vi "Monitor_Cliente_Consumidor.vi"() -> ()   [LabVIEW 2024]
uses:
  controls/Oven.ctl
  controls/Acquire.ctl
panel:
  out "# elements in queue":i32
  out "Temp Acq":string="View Acquired Data"
  out "State control":string="View Acquired Data"
  out "Ventilator":bool
  in  "User Control":T1
  out "Historic Data":T2
  out "Heater Lebel [V]":dbl
  in  "Quit":bool
  in  "Stop Acq":bool
  in  "Start Acq":bool
  out "Temp. Display":T3(graph)
  out "Temp [ºC]":dbl(slide) scale=0.0..100.0
  out "HEATER":string
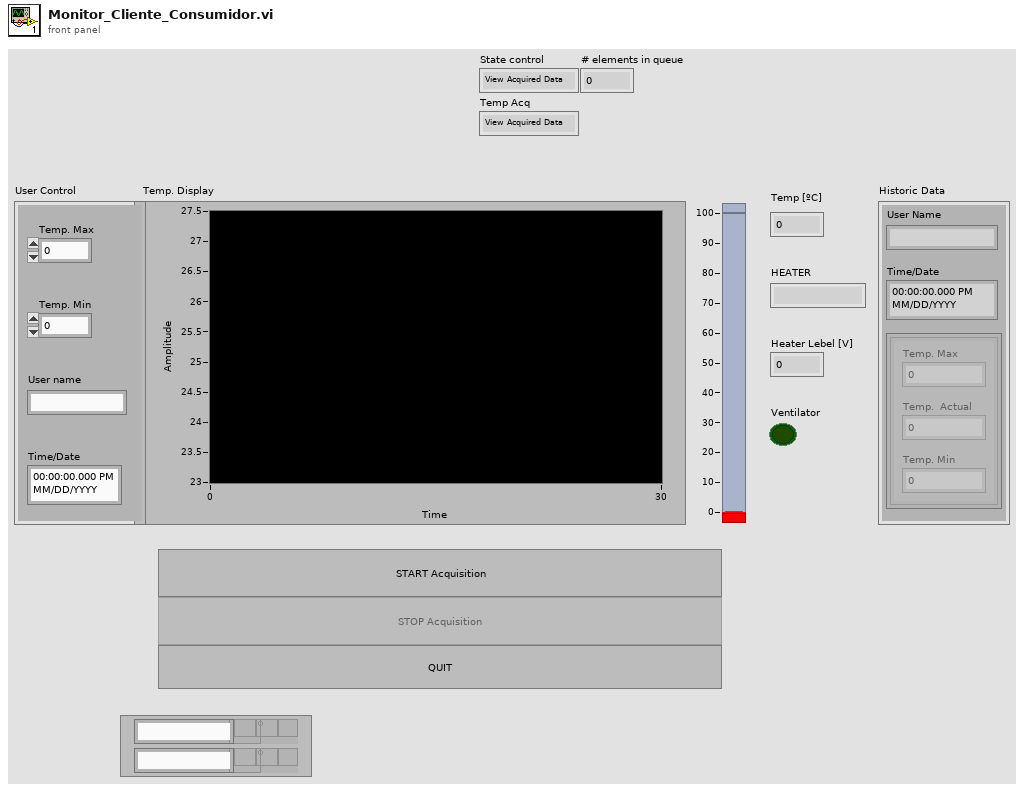
[diagram p1: front panel]
types:
  T1 = cluster{"Temp. Max":dbl, "Temp. Min":dbl, "User name":string, "Time/Date":timestamp}
  T2 = cluster{"User Name":string, "Time/Date":timestamp, "Array":cluster{"Temp. Max":dbl, "Temp.  Actual":dbl, "Temp. Min":dbl}[]}
  T3 = cluster{"Temp. Max":dbl, "Temp. Min":dbl, "RTD Temp":dbl}
  T4 = typedef "Acquire.ctl" = enum16{"Acquire", "Stop", "Exit", "Reset"}
  T5 = cluster{"RTD Temp":dbl, "Temp. Max":dbl, "Temp. Min":dbl}
  T6 = typedef "Oven.ctl" = enum16{"Initialize", "Measure", "Cooling", "Maximum", "Medium", "View Acquired Data", "Quit"}
  T7 = enum8{"Enabled", "Disabled", "Disabled and Grayed Out"}
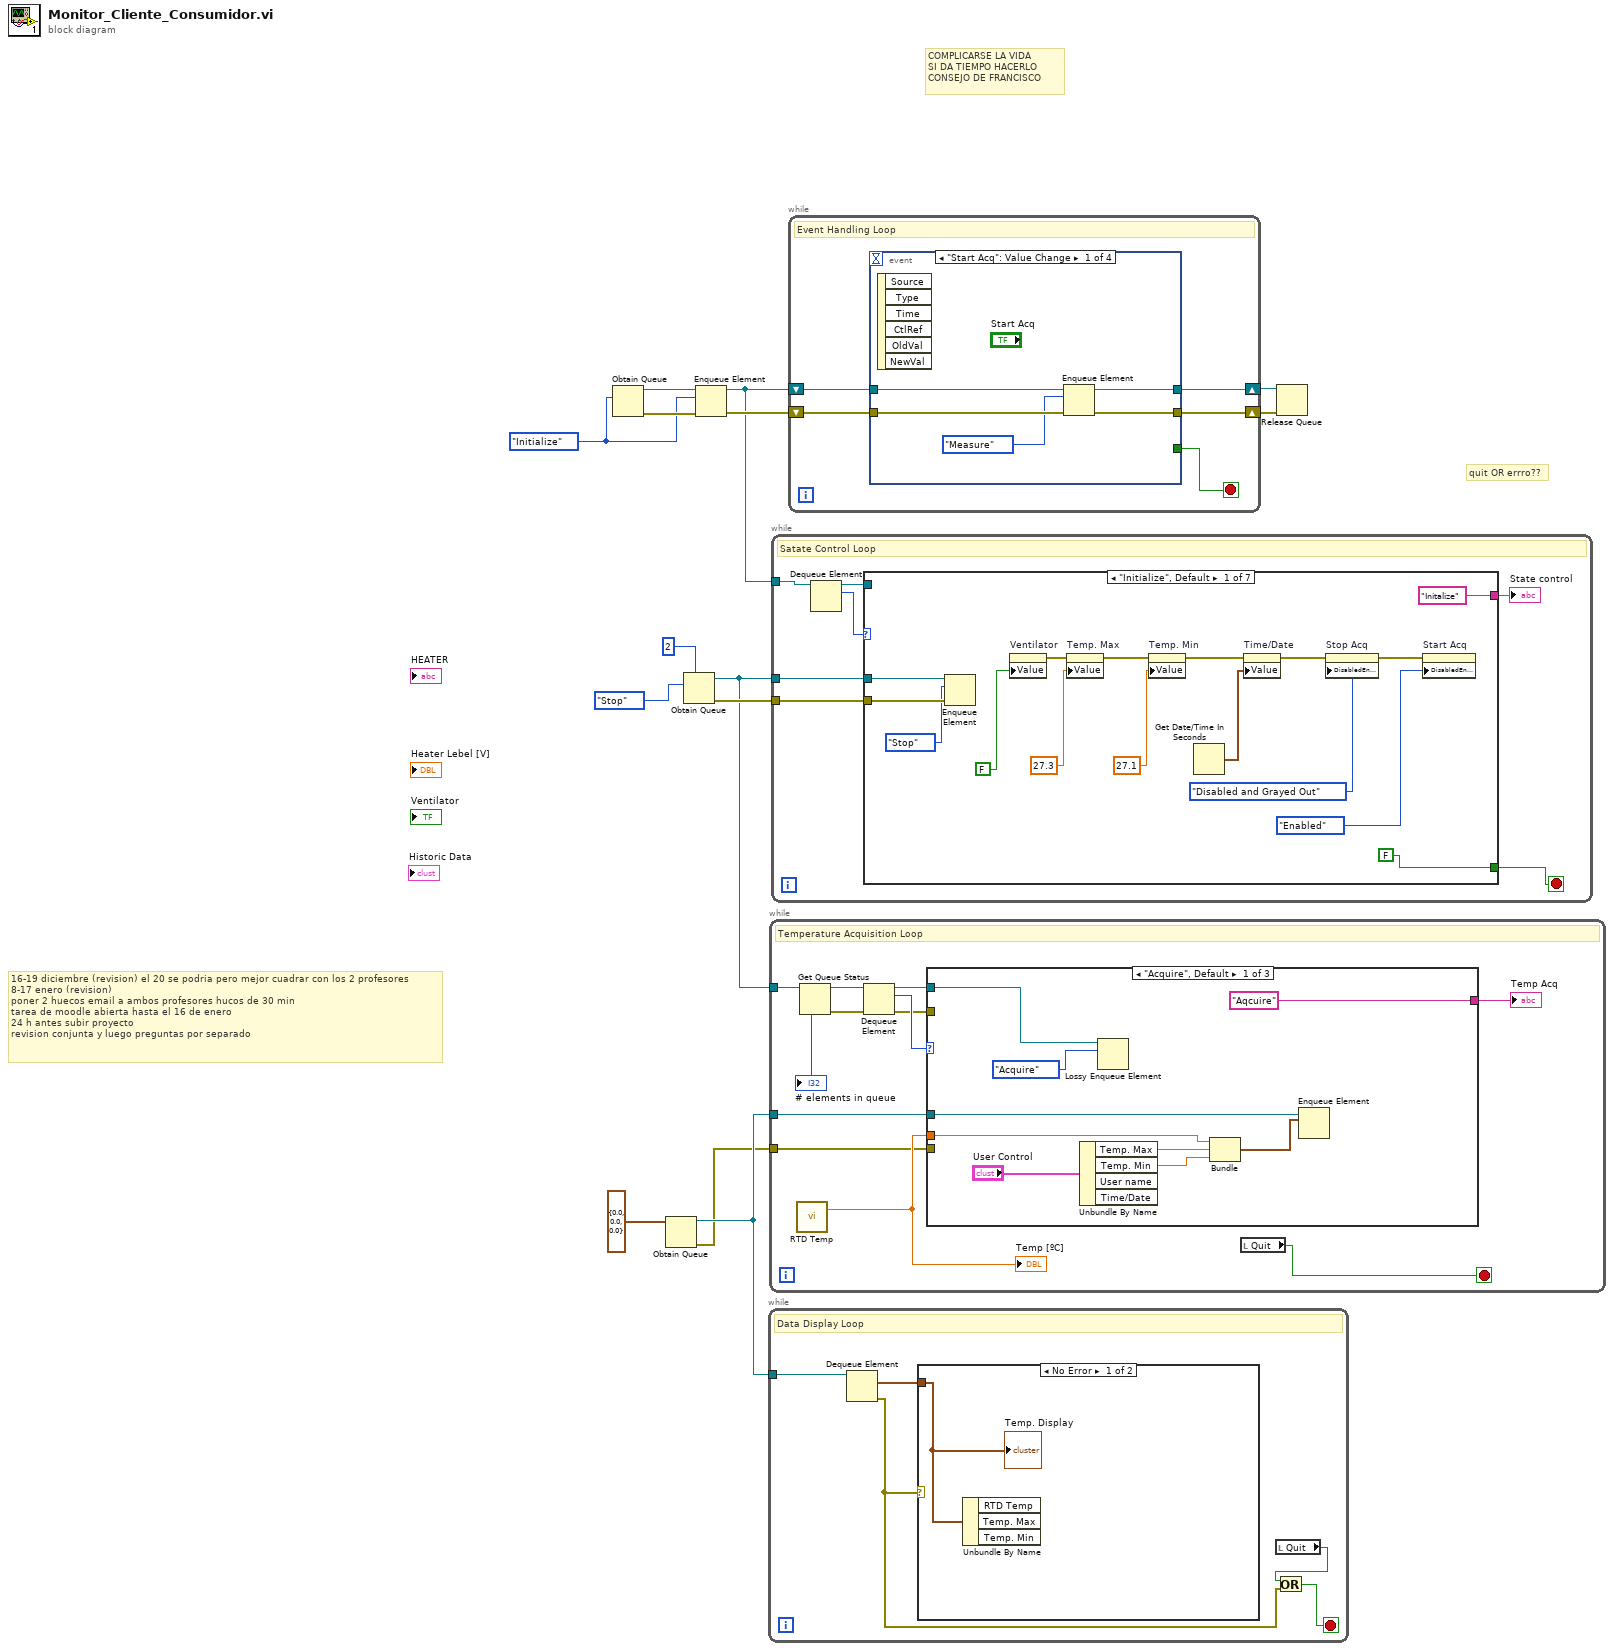
[diagram p0: block diagram]
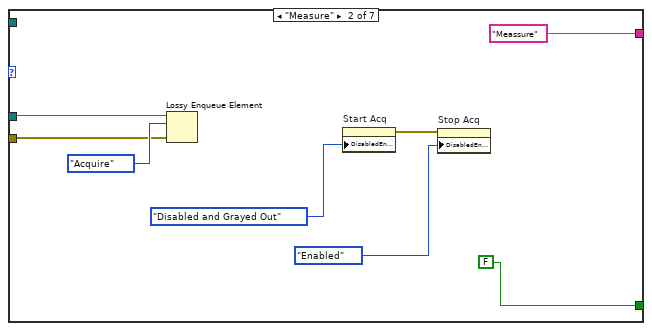
[diagram p2: hidden frame]
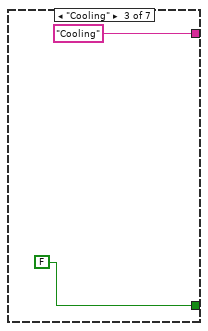
[diagram p3: hidden frame]
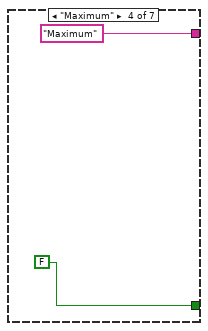
[diagram p4: hidden frame]
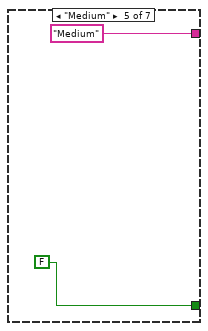
[diagram p5: hidden frame]
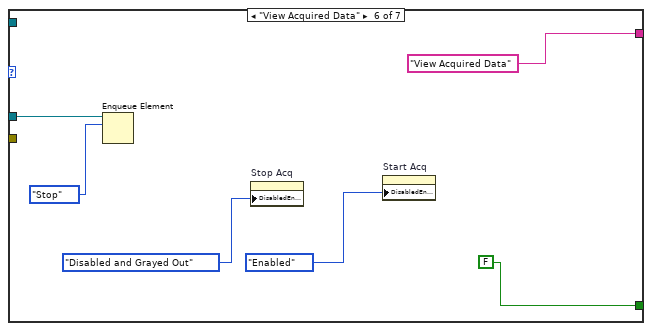
[diagram p6: hidden frame]
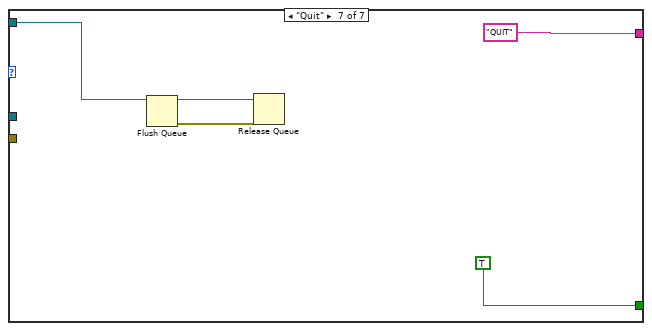
[diagram p7: hidden frame]
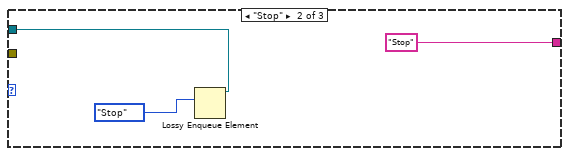
[diagram p8: hidden frame]
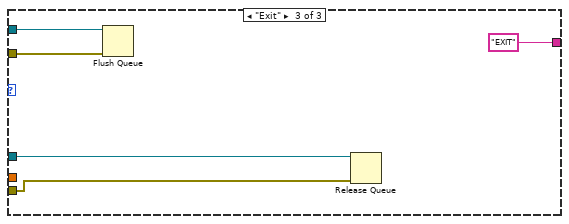
[diagram p9: hidden frame]
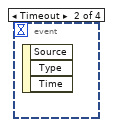
[diagram p10: hidden frame]
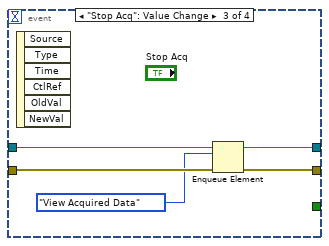
[diagram p11: hidden frame]
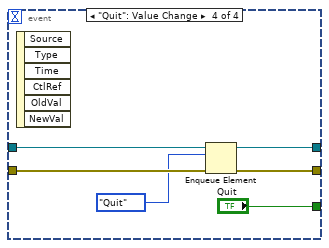
[diagram p12: hidden frame]
diagram:
  w6 = Oven."Initialize" ("Enum")
  # "COMPLICARSE LA VIDA \nSI DA TIEMPO HACERLO \nCONSEJO DE FRANCISCO"
  # "16-19 diciembre (revision) el 20 se podria pero mejor cuadrar con los 2 profesores \n8-17 enero (revision)\nponer 2 huecos email a ambos profesores hucos de 30 min\ntarea de moodle abierta hasta el 16 de enero\n24 h antes subir proyecto\nrevision conjunta y luego preguntas por separado"
  # "quit OR errro??"
  n1 = Obtain Queue(element data type=w6) -> (queue out=w8:refnum<queue>, error out=w9:errorcluster)  [unwired: 4 in, 1 out]
  n2 = Obtain Queue(element data type=T5 {"RTD Temp"=0.0, "Temp. Max"=0.0, "Temp. Min"=0.0} ("output cluster")) -> (queue out=w11:refnum<queue>, error out=w1:errorcluster)  [unwired: 4 in, 1 out]
  n3 = Obtain Queue(max queue size (-1, unlimited)=2, element data type=Acquire."Stop" ("Enum")) -> (queue out=w3:refnum<queue>, error out=w5:errorcluster)  [unwired: 3 in, 1 out]
  n4 = Enqueue Element(queue=w8, element=w6, error in (no error)=w9) -> (queue out=w7:refnum<queue>, error out=w10:errorcluster)  [unwired: 1 in, 1 out]
  n5 = while {
    tunnel: w11 -> [w18]
    stop <- w15 stop-if-true
    # "Data Display Loop"
    n6 = Dequeue Element(queue=w18) -> (element=w19:T5, error out=w16:errorcluster)  [unwired: 2 in, 2 out]
    n7 = case shown="No Error" w16 {
      tunnel: w19 -> [w20 _]
      frame No Error {
        n8 = Unbundle By Name(w20) -> ()  [unwired: 3 out]
        "Temp. Display" <- w20
      }
      frame Error {
      }
    }
    n9 = local read "Quit"() -> (w17:bool)
    n10 = Or(x=w17, y=w16) -> (x .or. y?=w15:bool)
  }
  n11 = while {
    tunnel: w11 -> [w30]
    tunnel: w3 -> [w27]
    tunnel: w1 -> [w23]
    stop <- w32 stop-if-true
    # "Temperature Acquisition Loop"
    n12 = call "RTD Temp.vi"() -> ("RTD Temp"=w28:dbl)  [unwired: 1 in, 1 out]
    "Temp [ºC]" <- w28
    n13 = Get Queue Status(queue=w27) -> (queue out=w25:refnum<queue>, error out=w22:errorcluster, # elements in queue=→"# elements in queue":i32)  [unwired: 2 in, 5 out]
    n14 = Dequeue Element(queue=w25, error in (no error)=w22) -> (queue out=w24:refnum<queue>, element=w31:T4, error out=w21:errorcluster)  [unwired: 1 in, 1 out]
    n15 = case shown="\"Acquire\", Default" w31 {
      tunnel: w30 -> [w38 _ w49]
      tunnel: ["Aqcuire" ("Temp Acq") "Stop" ("Temp Acq") "EXIT" ("Temp Acq")] -> w29
      tunnel: w28 -> [w35 _ _]
      tunnel: w24 -> [w33 w43 w46]
      tunnel: w23 -> [_ _ w48]
      tunnel: w21 -> [_ _ w45]
      frame "Acquire", Default {
        n16 = Unbundle By Name("User Control") -> ("Temp. Max"=w41:dbl, "Temp. Min"=w40:dbl)  [unwired: 2 out]
        n17 = Lossy Enqueue Element(queue=w33, element=Acquire."Acquire" ("Enum")) -> ()  [unwired: 1 in, 4 out]
        n18 = Bundle("RTD Temp"=w35, "Temp. Max"=w41, "Temp. Min"=w40) -> (w39:T5)  [unwired: 1 in]
        n19 = Enqueue Element(queue=w38, element=w39) -> ()  [unwired: 2 in, 3 out]
      }
      frame "Stop" {
        n20 = Lossy Enqueue Element(queue=w43, element=Acquire."Stop" ("Enum")) -> ()  [unwired: 1 in, 4 out]
      }
      frame "Exit" {
        n21 = Flush Queue(queue=w46, error in (no error)=w45) -> ()  [unwired: 3 out]
        n22 = Release Queue(queue=w49, error in (no error)=w48) -> ()  [unwired: 1 in, 3 out]
      }
    }
    "Temp Acq" <- w29
    n23 = local read "Quit"() -> (w32:bool)
  }
  n24 = while {
    tunnel: w7 -> [w56]
    tunnel: w3 -> [w54]
    tunnel: w5 -> [w53]
    stop <- w55 stop-if-true
    # "Satate Control Loop"
    n25 = Dequeue Element(queue=w56) -> (queue out=w50:refnum<queue>, element=w52:T6)  [unwired: 2 in, 2 out]
    n26 = case shown="\"Initialize\", Default" w52 {
      tunnel: [FALSE FALSE FALSE FALSE FALSE FALSE TRUE] -> w55
      tunnel: w54 -> [w59 w78 _ _ _ w90 _]
      tunnel: w53 -> [w58 w77 _ _ _ _ _]
      tunnel: ["Initalize" ("message") "Meassure" ("message") "Cooling" ("message") "Maximum" ("message") "Medium" ("message") "View Acquired Data" ("message") "QUIT" ("message")] -> w51
      tunnel: w50 -> [_ _ _ _ _ _ w94]
      frame "Initialize", Default {
        n27 = Enqueue Element(queue=w59, element=Acquire."Stop", error in (no error)=w58) -> ()  [unwired: 1 in, 3 out]
        n28 = property on="Ventilator" class="Bool (strict)"("Value"=FALSE ("Ventilator")) -> (error out=w64:errorcluster)  [unwired: 2 in, 1 out]
        n29 = property on="Temp. Max" class="DigNum (strict)"(error in=w64, "Value"=27.3) -> (error out=w69:errorcluster)  [unwired: 1 in, 1 out]
        n30 = property on="Temp. Min" class="DigNum (strict)"(error in=w69, "Value"=27.1) -> (error out=w67:errorcluster)  [unwired: 1 in, 1 out]
        n31 = Get Date/Time In Seconds() -> (seconds since 1Jan1904=w68:timestamp)
        n32 = property on="Time/Date" class="AbsTime (strict)"(error in=w67, "Value"=w68) -> (error out=w65:errorcluster)  [unwired: 1 in, 1 out]
        n33 = property on="Stop Acq" class="Bool (strict)"(error in=w65, "DisabledEnum"=T7."Disabled and Grayed Out" ("Disabled")) -> (error out=w60:errorcluster)  [unwired: 1 in, 1 out]
        n34 = property on="Start Acq" class="Bool (strict)"(error in=w60, "DisabledEnum"=T7."Enabled" ("Disabled")) -> ()  [unwired: 1 in, 2 out]
      }
      frame "Measure" {
        n35 = Lossy Enqueue Element(queue=w78, element=Acquire."Acquire" ("Enum"), error in (no error)=w77) -> ()  [unwired: 4 out]
        n36 = property on="Start Acq" class="Bool (strict)"("DisabledEnum"=T7."Disabled and Grayed Out" ("Disabled")) -> (error out=w75:errorcluster)  [unwired: 2 in, 1 out]
        n37 = property on="Stop Acq" class="Bool (strict)"(error in=w75, "DisabledEnum"=T7."Enabled" ("Disabled")) -> ()  [unwired: 1 in, 2 out]
      }
      frame "Cooling" {
      }
      frame "Maximum" {
      }
      frame "Medium" {
      }
      frame "View Acquired Data" {
        n38 = Enqueue Element(queue=w90, element=Acquire."Stop" ("Enum")) -> ()  [unwired: 2 in, 3 out]
        n39 = property on="Stop Acq" class="Bool (strict)"("DisabledEnum"=T7."Disabled and Grayed Out" ("Disabled")) -> ()  [unwired: 2 in, 2 out]
        n40 = property on="Start Acq" class="Bool (strict)"("DisabledEnum"=T7."Enabled" ("Disabled")) -> ()  [unwired: 2 in, 2 out]
      }
      frame "Quit" {
        n41 = Flush Queue(queue=w94) -> (queue out=w95:refnum<queue>, error out=w93:errorcluster)  [unwired: 1 in, 1 out]
        n42 = Release Queue(queue=w95, error in (no error)=w93) -> ()  [unwired: 1 in, 3 out]
      }
    }
    "State control" <- w51
  }
  n43 = while {
    shift-right: [w102] -> w14
    shift-left: w7 -> [w99]
    shift-right: [w101] -> w13
    shift-left: w10 -> [w100]
    stop <- w98 stop-if-true
    # "Event Handling Loop"
    n44 = event shown="[0] \"Start Acq\": Value Change" {
      selector: _ -> [_ _ _ _]
      dyn-events: _ -> [_ _ _ _]
      timeout: _ -> [_ _ _ _]
      tunnel: [w107 _ w111 w114] -> w102
      tunnel: [w106 _ w110 w115] -> w101
      tunnel: w100 -> [w105 _ w109 w116]
      tunnel: w99 -> [w104 _ w112 w117]
      tunnel: [_ _ _ "Quit"] -> w98
      event "Start Acq": Value Change {
        n45 = event-data() -> ()  [unwired: 1 in, 6 out]
        n46 = Enqueue Element(queue=w104, element=Oven."Measure", error in (no error)=w105) -> (queue out=w107:refnum<queue>, error out=w106:errorcluster)  [unwired: 1 in, 1 out]
      }
      event Timeout {
        n47 = event-data() -> ()  [unwired: 1 in, 3 out]
      }
      event "Stop Acq": Value Change {
        n48 = event-data() -> ()  [unwired: 1 in, 6 out]
        n49 = Enqueue Element(queue=w112, element=Oven."View Acquired Data", error in (no error)=w109) -> (queue out=w111:refnum<queue>, error out=w110:errorcluster)  [unwired: 1 in, 1 out]
      }
      event "Quit": Value Change {
        n50 = event-data() -> ()  [unwired: 1 in, 6 out]
        n51 = Enqueue Element(queue=w117, element=Oven."Quit", error in (no error)=w116) -> (queue out=w114:refnum<queue>, error out=w115:errorcluster)  [unwired: 1 in, 1 out]
      }
    }
  }
  n52 = Release Queue(queue=w14, error in (no error)=w13) -> ()  [unwired: 1 in, 3 out]
